vi "Interface_Asset_Map Control.vi"(8 "error in (no error)":errorcluster, 11 "EnergyStorage in":refnum<class "EnergyStorage.lvclass">) -> (0 "error out":errorcluster, 3 "EnergyStorage out":refnum<class "EnergyStorage.lvclass">)   [LabVIEW 2015, in "EnergyStorage.lvclass"]
uses:
  EnergyStorage.lvclass
  Interface_Asset/Interface_Asset.lvclass
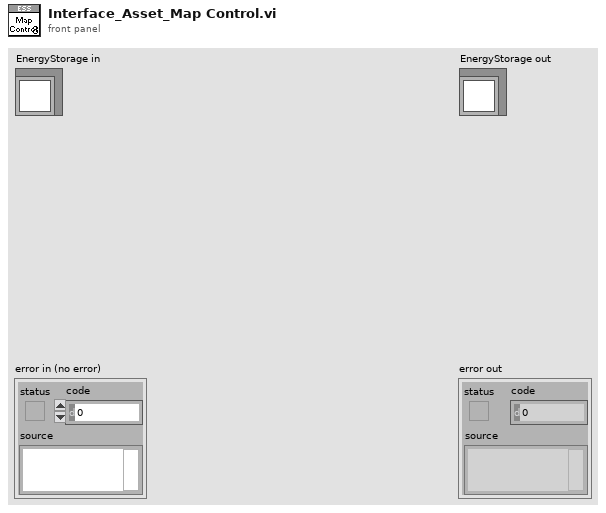
[diagram p1: front panel]
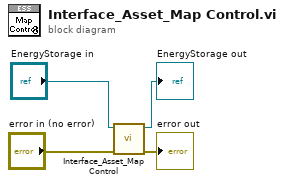
[diagram p0: block diagram]
diagram:
  n1 = call-parent "Interface_Asset_Map Control.vi"("error in (no error)"="error in (no error)", "Interface_Asset in"="EnergyStorage in") -> ("error out"=→"error out":errorcluster, "Interface_Asset out"=→"EnergyStorage out":refnum<class "EnergyStorage.lvclass">)  [unwired: 8 in]
